vi "bpms.vi"() -> ()   [LabVIEW 2015]
uses:
  <vilib>/Instr/_visa.llb/VISA Configure Serial Port (Instr).vi
panel:
  out "Discharge":bool[](array[boolean])
  out "0x41":string
  out "State of charge":dbl[](array[numeric]) format="%_3f%%"
  out "Voltage":dbl[](array[numeric]) format="%_4fV"
  out "Voltage":u16[](array[slide]) scale=26000.0..43000.0
  out "Temperature":u8[](array[numeric])
  out "0x69":string
  out "0x5A":string
  in  "VISA resource name":refnum<visa-resource-name>
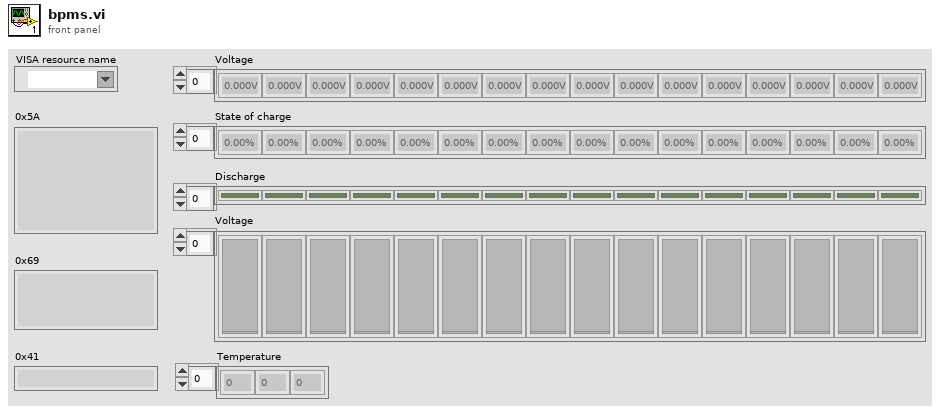
[diagram p1: front panel]
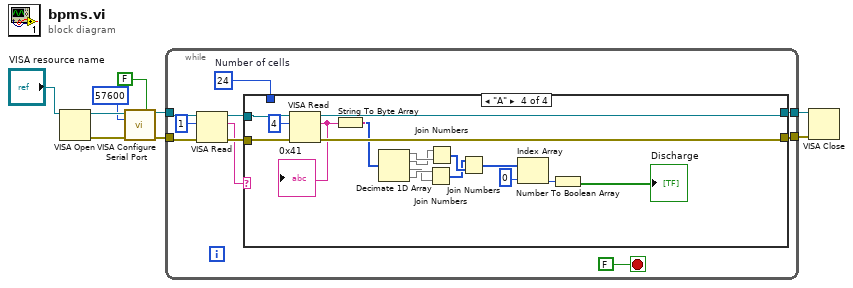
[diagram p0: block diagram]
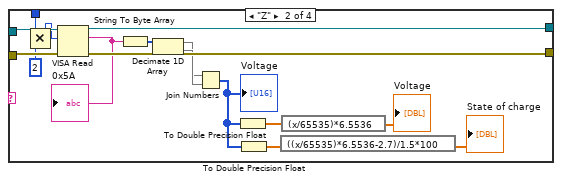
[diagram p3: hidden frame]
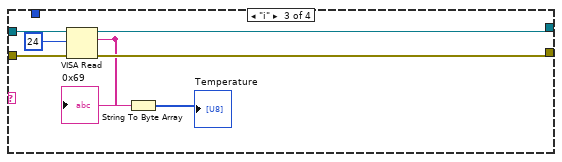
[diagram p4: hidden frame]
diagram:
  n1 = VISA Open(VISA resource name="VISA resource name") -> (VISA resource name=w8:refnum<visa-resource-name>, error out=w7:errorcluster)  [unwired: 4 in]
  n2 = call-poly "VISA Configure Serial Port"("VISA resource name"=w8, "Enable Termination\nChar (T)"=FALSE ("Enable Termination\nChar (T)"), "baud rate (9600)"=u32 57600, "error in (no error)"=w7) -> ("VISA resource name out"=w5:refnum<visa-resource-name>, "error out"=w4:errorcluster)  [unwired: 10 in]
  n3 = while {
    tunnel: w5 -> [w17]
    tunnel: w4 -> [w16]
    tunnel: [w13] -> w3
    tunnel: [w12] -> w2
    stop <- FALSE stop-if-true
    w10 = 24  # Number of cells
    n4 = VISA Read(VISA resource name=w17, byte count=u32 1, error in (no error)=w16) -> (VISA resource name out=w15:refnum<visa-resource-name>, read buffer=w11:string, error out=w14:errorcluster)  [unwired: 1 out]
    n5 = case shown="\"A\"" w11 {
      tunnel: w15 -> [w21 w26 w41 w60]
      tunnel: w14 -> [w20 w37 w42 w59]
      tunnel: [w21 w22 w44 w58] -> w13
      tunnel: [w20 w36 w43 w57] -> w12
      tunnel: w10 -> [_ w24 _ _]
      frame Default {
      }
      frame "Z" {
        n6 = Multiply(x=w24, y=2) -> (x*y=w25:i32)
        n7 = VISA Read(VISA resource name=w26, byte count=w25, error in (no error)=w37) -> (VISA resource name out=w22:refnum<visa-resource-name>, read buffer=w35:string, error out=w36:errorcluster)  [unwired: 1 out]
        "0x5A" <- w35
        n8 = String To Byte Array(string=w35) -> (unsigned byte array=w34:u8[])
        n9 = Decimate 1D Array(w34) -> (w32:u8[], w33:u8[])
        n10 = Join Numbers(hi=w32, lo=w33) -> ((hi.lo)=w27:u16[])
        "Voltage" <- w27
        n11 = To Double Precision Float(number=w27) -> (double precision float=w30:dbl[])
        n12 = To Double Precision Float(number=w27) -> (double precision float=w29:dbl[])
        n13 = expression code="((x/65535)*6.5536-2.7)/1.5*100"(w29) -> (→"State of charge":dbl[])
        n14 = expression code="(x/65535)*6.5536"(w30) -> (→"Voltage":dbl[])
      }
      frame "i" {
        n15 = VISA Read(VISA resource name=w41, byte count=u32 24, error in (no error)=w42) -> (VISA resource name out=w44:refnum<visa-resource-name>, read buffer=w40:string, error out=w43:errorcluster)  [unwired: 1 out]
        "0x69" <- w40
        n16 = String To Byte Array(string=w40) -> (unsigned byte array=→"Temperature":u8[])
      }
      frame "A" {
        n17 = VISA Read(VISA resource name=w60, byte count=u32 4, error in (no error)=w59) -> (VISA resource name out=w58:refnum<visa-resource-name>, read buffer=w56:string, error out=w57:errorcluster)  [unwired: 1 out]
        "0x41" <- w56
        n18 = String To Byte Array(string=w56) -> (unsigned byte array=w55:u8[])
        n19 = Decimate 1D Array(w55) -> (w51:u8[], w50:u8[], w48:u8[], w49:u8[])
        n20 = Join Numbers(hi=w49, lo=w48) -> ((hi.lo)=w45:u16[])
        n21 = Join Numbers(hi=w50, lo=w51) -> ((hi.lo)=w46:u16[])
        n22 = Join Numbers(hi=w45, lo=w46) -> ((hi.lo)=w47:u32[])
        n23 = Index Array(array=w47, index=0) -> (element=w53:u32)
        n24 = Number To Boolean Array(number=w53) -> (Boolean array=→"Discharge":bool[])
      }
    }
  }
  n25 = VISA Close(VISA resource name=w3, error in (no error)=w2) -> ()  [unwired: 1 out]
